vi "New Resource from UTF-16 Item.vi"(7 "Shared? (f)":bool, 8 "error in (no error)":errorcluster, 9 "Default String (UTF-16)":string, 10 "Tag (ANSI)":string, 11 "LangFile in":refnum<class "Resource Data.lvclass">) -> (0 "error out":errorcluster, 2 "RID":string, 3 "LangFile out":refnum<class "Resource Data.lvclass">)   [LabVIEW 2013, in "SET Project Data.lvlib" / "Resource Data.lvclass"]
uses:
  Resource Data.lvclass
  Types/ProjFile_Resource Entry.ctl
  Resource Data.lvclass/Resource Data.ctl
  Read Languages.vi
  SET Project Data.lvlib
panel:
  # "- Generate new RID\n- Add entry to resource table"
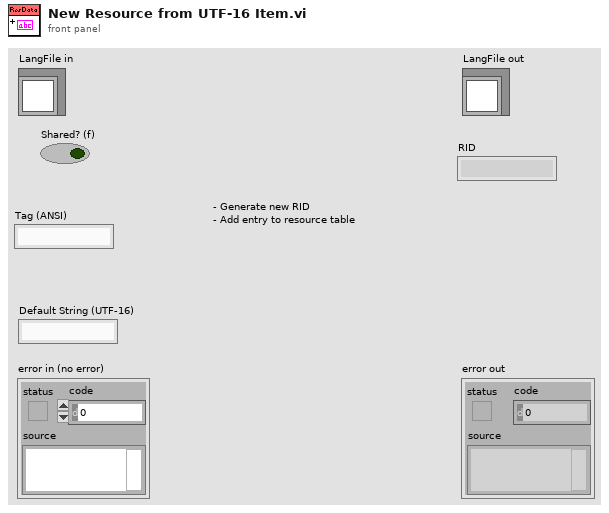
[diagram p1: front panel]
types:
  T1 = typedef "SET Project Data.lvlib/ProjFile_Resource Entry.ctl" = cluster{"RID":string, "Tag":string, "Strings [] (UTF-16)":string[], "Shared?":bool}
  T2 = typedef "SET Project Data.lvlib/ProjFile_Language Data.ctl" = cluster{"Tag":string, "Name":string, "Code Page":u16}
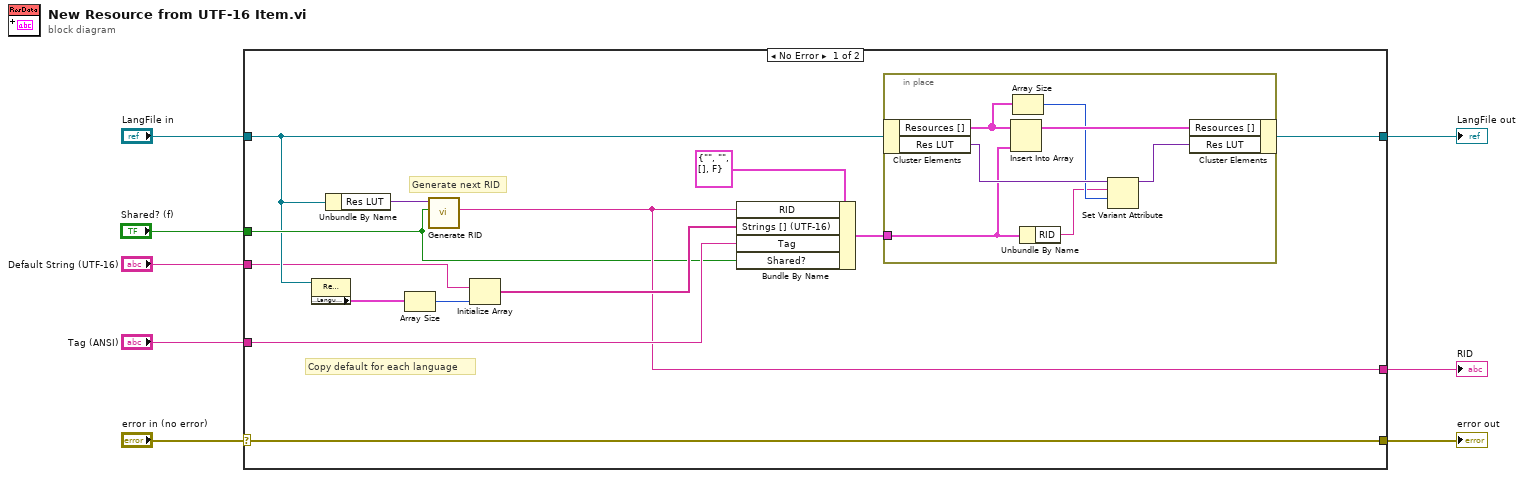
[diagram p0: block diagram]
diagram:
  n1 = case shown="No Error" "error in (no error)" {
    selector: "error in (no error)" -> [w21 w30]
    tunnel: [w21 w30] -> w7
    tunnel: [w18 w29] -> w5
    tunnel: "LangFile in" -> [w11 w29]
    tunnel: "Shared? (f)" -> [w12 _]
    tunnel: "Tag (ANSI)" -> [w15 _]
    tunnel: "Default String (UTF-16)" -> [w9 _]
    tunnel: [w13 _] -> w1
    frame No Error {
      # "Copy default for each language"
      # "Generate next RID"
      n2 = property class="Resource Data.lvclass"(reference=w11) -> ("Properties:Languages []"=w10:T2[])  [unwired: 1 in, 2 out]
      n3 = Unbundle By Name(w11) -> ("Res LUT"=w14:variant)
      n4 = Array Size(array=w10) -> (size(s)=w20:i32)
      n5 = call "Generate RID.vi"("Negative? (F)"=w12, "LUT in"=w14) -> ("Unique Key"=w13:string)  [unwired: 8 in, 1 out]
      n6 = Initialize Array(w9, w20) -> (w16:string[])
      n7 = Bundle By Name(cluster=T1 {"RID"="", "Tag"="", "Strings [] (UTF-16)"=[], "Shared?"=FALSE} ("Resource"), "RID"=w13, "Strings [] (UTF-16)"=w16, "Tag"=w15, "Shared?"=w12) -> (w17:T1)
      n8 = in-place {
        in-place-border: w17 -> [w23]
        n9 = in-place-cluster #1(w11) -> ("Resources []"=w25:T1[], "Res LUT"=w27:variant)
        n10 = Insert Into Array(array=w25, new element=w23) -> (w28:T1[])  [unwired: 1 in]
        n11 = Array Size(array=w25) -> (size(s)=w24:i32)
        n12 = Unbundle By Name(w23) -> ("RID"=w22:string)
        n13 = Set Variant Attribute(Variant=w27, name=w22, value=w24) -> (Variant out=w26:variant)  [unwired: 1 in, 2 out]
        n14 = in-place-cluster #1("Resources []"=w28, "Res LUT"=w26) -> (w18:refnum<class "Resource Data.lvclass">)
      }
    }
    frame Error {
    }
  }
  "error out" <- w7
  "LangFile out" <- w5
  "RID" <- w1
